vi "LC Transfer.vi"(8 "error in (no error)":errorcluster caption="Error In", 9 "Value In":string, 10 "Property":string, 11 "Ctl Ref In":refnum<vi>) -> (0 "error out":errorcluster caption="Error Out", 1 "Value Out":string, 3 "Ctl Ref Out":refnum<vi>)   [LabVIEW 2020]
uses:
  <vilib>/Utility/miscctls.llb/LVOutOfRangeActionTypeDef.ctl
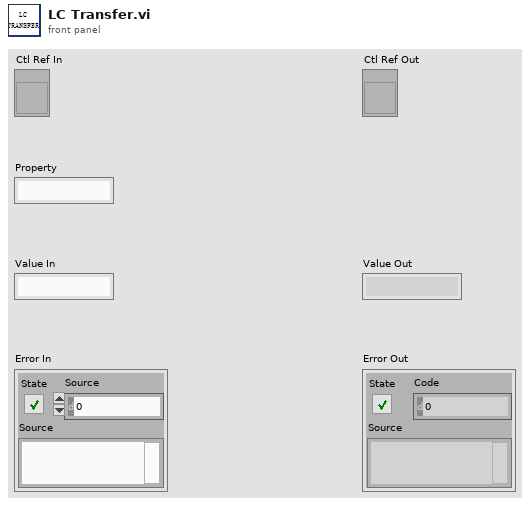
[diagram p1: front panel]
types:
  T1 = typedef "LVPositionTypeDef.ctl" = cluster{"Left":i32, "Top":i32}
  T2 = typedef "LVOutOfRangeActionTypeDef.ctl" = cluster{"Out of Range Action Minimum":u8, "Out of Range Action Maximum":u8, "Out of Range Action Increment":u8}
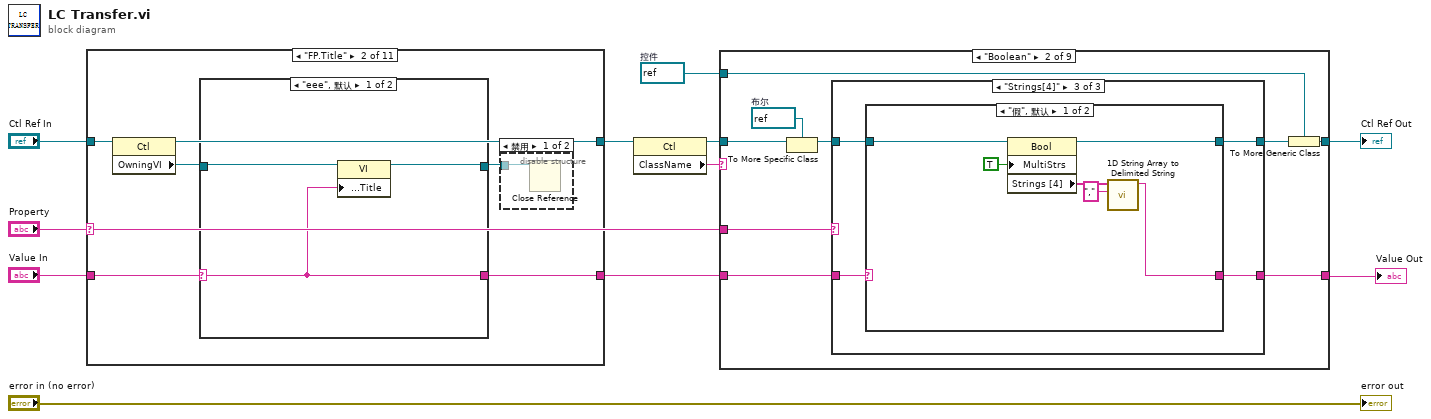
[diagram p0: block diagram]
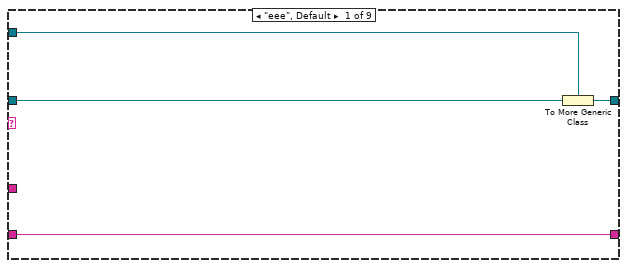
[diagram p2: hidden frame]
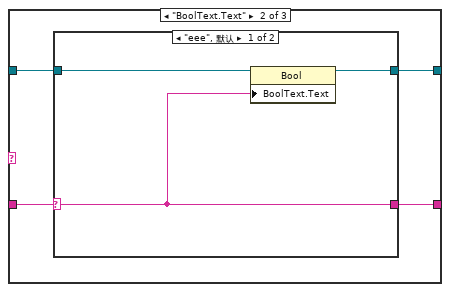
[diagram p4: hidden frame]
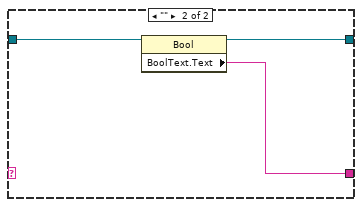
[diagram p5: hidden frame]
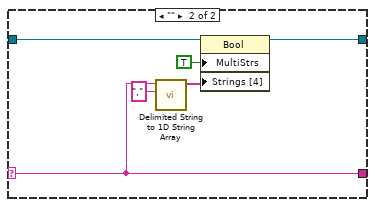
[diagram p6: hidden frame]
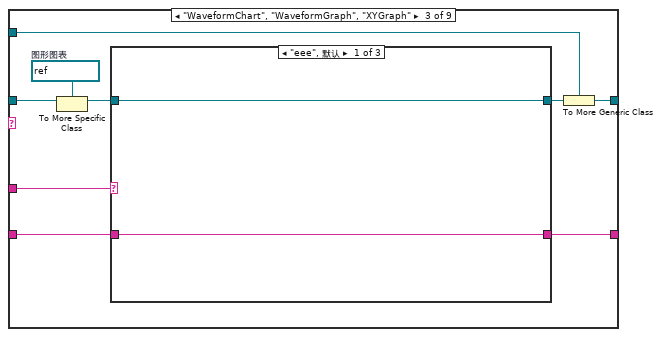
[diagram p7: hidden frame]
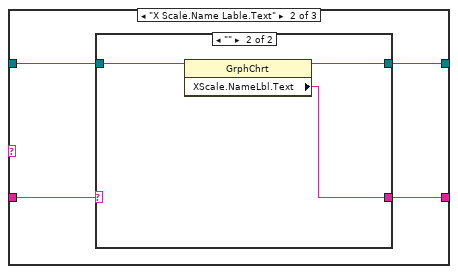
[diagram p8: hidden frame]
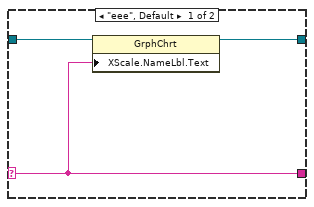
[diagram p9: hidden frame]
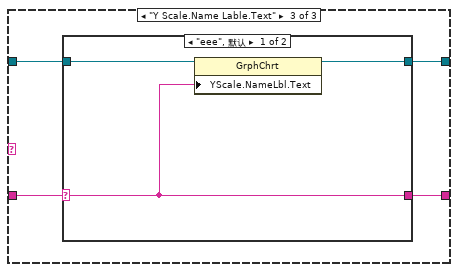
[diagram p10: hidden frame]
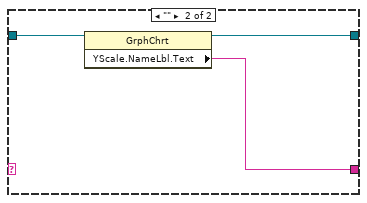
[diagram p11: hidden frame]
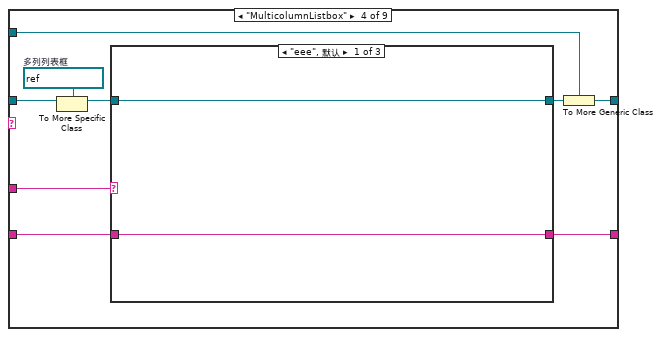
[diagram p12: hidden frame]
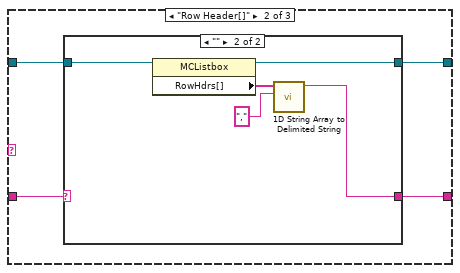
[diagram p13: hidden frame]
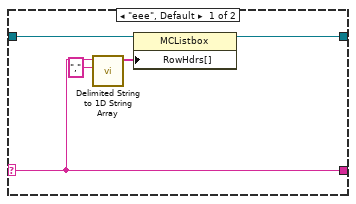
[diagram p14: hidden frame]
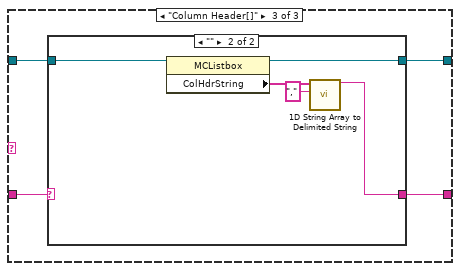
[diagram p15: hidden frame]
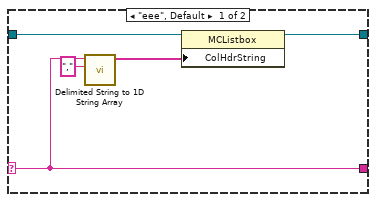
[diagram p16: hidden frame]
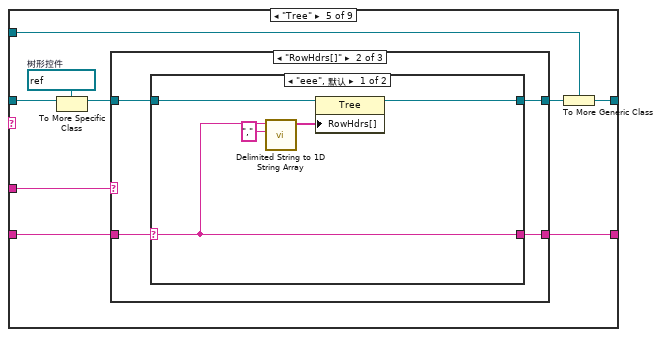
[diagram p17: hidden frame]
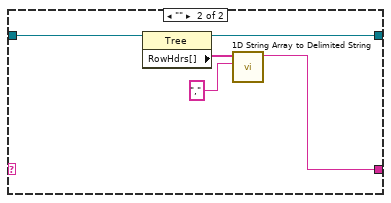
[diagram p19: hidden frame]
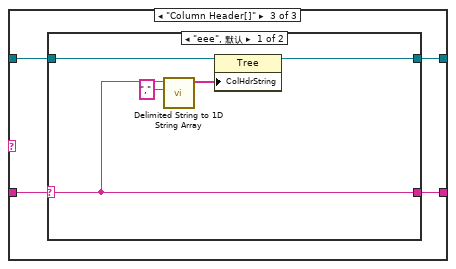
[diagram p20: hidden frame]
diagram:
  w10 = refnum<vi> refnum  # 控件
  n1 = case shown="\"FP.Title\"" "Property" {
    tunnel: [w13 w18 w27 w38 w48 w59 w75 w91 w107 w123 w146] -> w11
    tunnel: "Ctl Ref In" -> [w13 w19 w29 w40 w50 w60 w76 w92 w108 w124 w147]
    tunnel: "Value In" -> [w12 w15 w30 w39 w49 w58 w74 w90 w106 w122 w145]
    tunnel: [w12 w14 w28 w37 w47 w57 w73 w89 w105 w121 w144] -> w9
    frame "eee", Default {
    }
    frame "FP.Title" {
      n2 = property class="Ctl"(reference=w19) -> (reference out=w18:refnum<vi>, "OwningVI"=w17:refnum<vi>)  [unwired: 1 in, 1 out]
      n3 = case shown="\"eee\", 默认" w15 {
        selector: w15 -> [w21 _]
        tunnel: w17 -> [w23 w26]
        tunnel: [w22 w25] -> w16
        tunnel: [w21 w24] -> w14
        frame "eee", Default {
          n4 = property class="VI"(reference=w23, "Front Panel.Title"=w21) -> (reference out=w22:refnum<vi>)  [unwired: 1 in, 1 out]
        }
        frame "" {
          n5 = property class="VI"(reference=w26) -> (reference out=w25:refnum<vi>, "Front Panel.Title"=w24:string)  [unwired: 1 in, 1 out]
        }
      }
      n6 = disable-structure shown="禁用" {
        disable-tunnel: w16 -> [w20 _]
        frame Disabled {
          n7 = Close Reference(reference=w20) -> ()  [unwired: 1 in, 1 out]
        }
        frame Enabled {
        }
      }
    }
    frame "Lable.Text" {
      n8 = case shown="\"eee\", 默认" w30 {
        selector: w30 -> [w31 _]
        tunnel: w29 -> [w33 w36]
        tunnel: [w31 w35] -> w28
        tunnel: [w32 w34] -> w27
        frame "eee", Default {
          n9 = property class="Ctl"(reference=w33, "Label.Text"=w31) -> (reference out=w32:refnum<vi>)  [unwired: 1 in, 1 out]
        }
        frame "" {
          n10 = property class="Ctl"(reference=w36) -> (reference out=w34:refnum<vi>, "Label.Text"=w35:string)  [unwired: 1 in, 1 out]
        }
      }
    }
    frame "Desc" {
      n11 = case shown="\"eee\", 默认" w39 {
        selector: w39 -> [w41 _]
        tunnel: w40 -> [w43 w46]
        tunnel: [w42 w45] -> w38
        tunnel: [w41 w44] -> w37
        frame "eee", Default {
          n12 = property class="Ctl"(reference=w43, "Desc"=w41) -> (reference out=w42:refnum<vi>)  [unwired: 1 in, 1 out]
        }
        frame "" {
          n13 = property class="Ctl"(reference=w46) -> (reference out=w45:refnum<vi>, "Desc"=w44:string)  [unwired: 1 in, 1 out]
        }
      }
    }
    frame "TipStrip" {
      n14 = case shown="\"eee\", 默认" w49 {
        selector: w49 -> [w51 _]
        tunnel: w50 -> [w53 w56]
        tunnel: [w52 w55] -> w48
        tunnel: [w51 w54] -> w47
        frame "eee", Default {
          n15 = property class="Ctl"(reference=w53, "TipStrip"=w51) -> (reference out=w52:refnum<vi>)  [unwired: 1 in, 1 out]
        }
        frame "" {
          n16 = property class="Ctl"(reference=w56) -> (reference out=w55:refnum<vi>, "TipStrip"=w54:string)  [unwired: 1 in, 1 out]
        }
      }
    }
    frame "Visible" {
      n17 = case shown="\"eee\", 默认" w58 {
        selector: w58 -> [_ w67]
        tunnel: w60 -> [w66 w72]
        tunnel: [w65 w71] -> w59
        tunnel: [w61 w67] -> w57
        frame "eee", Default {
          n18 = property class="Ctl"(reference=w66) -> (reference out=w65:refnum<vi>, "Visible"=w64:bool)  [unwired: 1 in, 1 out]
          n19 = Select(t="1", s=w64, f="0") -> (s? t:f=w61:string)
        }
        frame "" {
          n20 = call <vilib>:"Trim Whitespace.vi"("string"=w67) -> ("trimmed string"=w70:string)  [unwired: 1 in]
          n21 = Decimal String To Number(string=w70) -> (number=w69:i32)  [unwired: 2 in, 1 out]
          n22 = Greater Than 0?(x=w69) -> (x > 0?=w68:bool)
          n23 = property class="Ctl"(reference=w72, "Visible"=w68) -> (reference out=w71:refnum<vi>)  [unwired: 1 in, 1 out]
        }
      }
    }
    frame "Caption.Visible" {
      n24 = case shown="\"eee\", 默认" w74 {
        selector: w74 -> [w77 _]
        tunnel: w76 -> [w82 w88]
        tunnel: [w81 w83] -> w75
        tunnel: [w77 w84] -> w73
        frame "eee", Default {
          n25 = call <vilib>:"Trim Whitespace.vi"("string"=w77) -> ("trimmed string"=w80:string)  [unwired: 1 in]
          n26 = Decimal String To Number(string=w80) -> (number=w79:i32)  [unwired: 2 in, 1 out]
          n27 = Greater Than 0?(x=w79) -> (x > 0?=w78:bool)
          n28 = property class="Ctl"(reference=w82, "Caption.Visible"=w78) -> (reference out=w81:refnum<vi>)  [unwired: 1 in, 1 out]
        }
        frame "" {
          n29 = property class="Ctl"(reference=w88) -> (reference out=w83:refnum<vi>, "Caption.Visible"=w87:bool)  [unwired: 1 in, 1 out]
          n30 = Select(t="1", s=w87, f="0") -> (s? t:f=w84:string)
        }
      }
    }
    frame "Lable.Visible" {
      n31 = case shown="\"eee\", 默认" w90 {
        selector: w90 -> [w93 _]
        tunnel: w92 -> [w98 w104]
        tunnel: [w97 w99] -> w91
        tunnel: [w93 w100] -> w89
        frame "eee", Default {
          n32 = call <vilib>:"Trim Whitespace.vi"("string"=w93) -> ("trimmed string"=w96:string)  [unwired: 1 in]
          n33 = Decimal String To Number(string=w96) -> (number=w95:i32)  [unwired: 2 in, 1 out]
          n34 = Greater Than 0?(x=w95) -> (x > 0?=w94:bool)
          n35 = property class="Ctl"(reference=w98, "Label.Visible"=w94) -> (reference out=w97:refnum<vi>)  [unwired: 1 in, 1 out]
        }
        frame "" {
          n36 = property class="Ctl"(reference=w104) -> (reference out=w99:refnum<vi>, "Label.Visible"=w103:bool)  [unwired: 1 in, 1 out]
          n37 = Select(t="1", s=w103, f="0") -> (s? t:f=w100:string)
        }
      }
    }
    frame "Blinking" {
      n38 = case shown="\"eee\", 默认" w106 {
        selector: w106 -> [w109 _]
        tunnel: w108 -> [w114 w120]
        tunnel: [w113 w119] -> w107
        tunnel: [w109 w115] -> w105
        frame "eee", Default {
          n39 = call <vilib>:"Trim Whitespace.vi"("string"=w109) -> ("trimmed string"=w112:string)  [unwired: 1 in]
          n40 = Decimal String To Number(string=w112) -> (number=w111:i32)  [unwired: 2 in, 1 out]
          n41 = Greater Than 0?(x=w111) -> (x > 0?=w110:bool)
          n42 = property class="Ctl"(reference=w114, "Blinking"=w110) -> (reference out=w113:refnum<vi>)  [unwired: 1 in, 1 out]
        }
        frame "" {
          n43 = property class="Ctl"(reference=w120) -> (reference out=w119:refnum<vi>, "Blinking"=w118:bool)  [unwired: 1 in, 1 out]
          n44 = Select(t="1", s=w118, f="0") -> (s? t:f=w115:string)
        }
      }
    }
    frame "Caption.Position" {
      n45 = case shown="\"\"" w122 {
        selector: w122 -> [w125 _]
        tunnel: w124 -> [w133 w143]
        tunnel: [w132 w134] -> w123
        tunnel: [w125 w135] -> w121
        frame "eee", Default {
          n46 = call <vilib>:"Delimited String to 1D String Array.vi"("delimiter"=",", "delimited string"=w125) -> ("string array"=w130:string[])  [unwired: 9 in]
          n47 = Fract/Exp String To Number(string=w130) -> (number=w129:dbl[])  [unwired: 3 in, 1 out]
          n48 = Index Array(array=w129) -> (element #1=w128:dbl, element #2=w127:dbl)  [unwired: 2 in]
          n49 = Bundle("String"=w128, "String"=w127) -> (w126:cluster{"String":dbl, "String":dbl})  [unwired: 1 in]
          n50 = property class="Ctl"(reference=w133, "Caption.Position"=w126) -> (reference out=w132:refnum<vi>)  [unwired: 1 in, 1 out]
        }
        frame "" {
          n51 = property class="Ctl"(reference=w143) -> (reference out=w134:refnum<vi>, "Caption.Position"=w142:T1)  [unwired: 1 in, 1 out]
          n52 = Unbundle(w142) -> ("Left"=w141:i32, "Top"=w140:i32)
          n53 = Build Array(w141, w140) -> (w139:i32[])
          n54 = Number To Fractional String(number=w139, precision (6)=i16 0 ("精度(6)")) -> (F-format string=w137:string[])  [unwired: 2 in]
          n55 = call <vilib>:"1D String Array to Delimited String.vi"("delimiter"=",", "string array"=w137) -> ("delimited string"=w135:string)  [unwired: 9 in]
        }
      }
    }
    frame "Caption.Text" {
      n56 = case shown="\"eee\", 默认" w145 {
        selector: w145 -> [w148 _]
        tunnel: w147 -> [w152 w155]
        tunnel: [w151 w154] -> w146
        tunnel: [w148 w153] -> w144
        frame "eee", Default {
          n57 = property class="Ctl"(reference=w152, "Caption.Visible"=TRUE ("可见"), "Caption.Text"=w148, "Label.Visible"=FALSE ("标签.可见")) -> (reference out=w151:refnum<vi>)  [unwired: 1 in, 1 out]
        }
        frame "" {
          n58 = property class="Ctl"(reference=w155, "Visible"=TRUE ("可见")) -> (reference out=w154:refnum<vi>, "Caption.Text"=w153:string)  [unwired: 1 in, 1 out]
        }
      }
    }
  }
  n59 = property class="Ctl"(reference=w11) -> (reference out=w4:refnum<vi>, "ClassName"=w3:string)  [unwired: 1 in, 1 out]
  n60 = case shown="\"Boolean\"" w3 {
    tunnel: "Property" -> [_ w169 w205 w236 w275 w314 w339 w387 w433]
    tunnel: w4 -> [w160 w168 w206 w237 w276 w315 w340 w389 w434]
    tunnel: [w159 w164 w204 w235 w274 w313 w338 w383 w430] -> w5
    tunnel: w10 -> [w158 w163 w203 w234 w273 w312 w337 w382 _]
    tunnel: w9 -> [w157 w162 w199 w230 w270 w308 w333 w384 w432]
    tunnel: [w157 w161 w198 w229 w268 w307 w332 w381 w429] -> w2
    frame "eee", Default {
      n61 = To More Generic Class(target class=w158, reference=w160) -> (generic class reference=w159:refnum<vi>)
    }
    frame "Boolean" {
      w166 = refnum<vi> refnum  # 布尔
      n62 = To More Specific Class(target class=w166, reference=w168) -> (specific class reference=w167:refnum<vi>)  [unwired: 1 in, 1 out]
      n63 = case shown="\"Strings[4]\"" w169 {
        tunnel: w167 -> [w171 w175 w185]
        tunnel: [w171 w174 w184] -> w165
        tunnel: w162 -> [w170 w173 w183]
        tunnel: [w170 w172 w182] -> w161
        frame "eee", Default {
        }
        frame "BoolText.Text" {
          n64 = case shown="\"eee\", 默认" w173 {
            selector: w173 -> [w176 _]
            tunnel: w175 -> [w178 w181]
            tunnel: [w177 w180] -> w174
            tunnel: [w176 w179] -> w172
            frame "eee", Default {
              n65 = property class="Bool"(reference=w178, "BoolText.Text"=w176) -> (reference out=w177:refnum<vi>)  [unwired: 1 in, 1 out]
            }
            frame "" {
              n66 = property class="Bool"(reference=w181) -> (reference out=w180:refnum<vi>, "BoolText.Text"=w179:string)  [unwired: 1 in, 1 out]
            }
          }
        }
        frame "Strings[4]" {
          n67 = case shown="\"假\", 默认" w183 {
            selector: w183 -> [_ w192]
            tunnel: w185 -> [w191 w196]
            tunnel: [w190 w195] -> w184
            tunnel: [w186 w192] -> w182
            frame "假", Default {
              n68 = property class="Bool"(reference=w191, "MultiStrs"=TRUE ("多文本字符串")) -> (reference out=w190:refnum<vi>, "Strings [4]"=w188:string[])  [unwired: 1 in, 1 out]
              n69 = call <vilib>:"1D String Array to Delimited String.vi"("delimiter"=",", "string array"=w188) -> ("delimited string"=w186:string)  [unwired: 9 in]
            }
            frame "" {
              n70 = call <vilib>:"Delimited String to 1D String Array.vi"("delimiter"=",", "delimited string"=w192) -> ("string array"=w193:string[])  [unwired: 9 in]
              n71 = property class="Bool"(reference=w196, "MultiStrs"=TRUE ("多文本字符串"), "Strings [4]"=w193) -> (reference out=w195:refnum<vi>)  [unwired: 1 in, 1 out]
            }
          }
        }
      }
      n72 = To More Generic Class(target class=w163, reference=w165) -> (generic class reference=w164:refnum<vi>)
    }
    frame "WaveformChart", "WaveformGraph", "XYGraph" {
      w200 = refnum<vi> refnum  # 图形图表
      n73 = To More Specific Class(target class=w200, reference=w206) -> (specific class reference=w202:refnum<vi>)  [unwired: 1 in, 1 out]
      n74 = case shown="\"eee\", 默认" w205 {
        tunnel: w202 -> [w208 w212 w222]
        tunnel: [w208 w211 w221] -> w201
        tunnel: w199 -> [w207 w210 w220]
        tunnel: [w207 w209 w219] -> w198
        frame "eee", Default {
        }
        frame "X Scale.Name Lable.Text" {
          n75 = case shown="\"\"" w210 {
            selector: w210 -> [w213 _]
            tunnel: w212 -> [w215 w218]
            tunnel: [w214 w217] -> w211
            tunnel: [w213 w216] -> w209
            frame "eee", Default {
              n76 = property class="GrphChrt"(reference=w215, "XScale.NameLbl.Text"=w213) -> (reference out=w214:refnum<vi>)  [unwired: 1 in, 1 out]
            }
            frame "" {
              n77 = property class="GrphChrt"(reference=w218) -> (reference out=w217:refnum<vi>, "XScale.NameLbl.Text"=w216:string)  [unwired: 1 in, 1 out]
            }
          }
        }
        frame "Y Scale.Name Lable.Text" {
          n78 = case shown="\"eee\", 默认" w220 {
            selector: w220 -> [w223 _]
            tunnel: w222 -> [w225 w228]
            tunnel: [w224 w227] -> w221
            tunnel: [w223 w226] -> w219
            frame "eee", Default {
              n79 = property class="GrphChrt"(reference=w225, "YScale.NameLbl.Text"=w223) -> (reference out=w224:refnum<vi>)  [unwired: 1 in, 1 out]
            }
            frame "" {
              n80 = property class="GrphChrt"(reference=w228) -> (reference out=w227:refnum<vi>, "YScale.NameLbl.Text"=w226:string)  [unwired: 1 in, 1 out]
            }
          }
        }
      }
      n81 = To More Generic Class(target class=w203, reference=w201) -> (generic class reference=w204:refnum<vi>)
    }
    frame "MulticolumnListbox" {
      w231 = refnum<vi> refnum  # 多列列表框
      n82 = To More Specific Class(target class=w231, reference=w237) -> (specific class reference=w233:refnum<vi>)  [unwired: 1 in, 1 out]
      n83 = case shown="\"eee\", 默认" w236 {
        tunnel: w233 -> [w239 w243 w257]
        tunnel: [w239 w242 w256] -> w232
        tunnel: w230 -> [w238 w241 w255]
        tunnel: [w238 w240 w254] -> w229
        frame "eee", Default {
        }
        frame "Row Header[]" {
          n84 = case shown="\"\"" w241 {
            selector: w241 -> [w244 _]
            tunnel: w243 -> [w248 w253]
            tunnel: [w247 w252] -> w242
            tunnel: [w244 w249] -> w240
            frame "eee", Default {
              n85 = call <vilib>:"Delimited String to 1D String Array.vi"("delimiter"=",", "delimited string"=w244) -> ("string array"=w245:string[])  [unwired: 9 in]
              n86 = property class="MCListbox"(reference=w248, "RowHdrs[]"=w245) -> (reference out=w247:refnum<vi>)  [unwired: 1 in, 1 out]
            }
            frame "" {
              n87 = property class="MCListbox"(reference=w253) -> (reference out=w252:refnum<vi>, "RowHdrs[]"=w251:string[])  [unwired: 1 in, 1 out]
              n88 = call <vilib>:"1D String Array to Delimited String.vi"("delimiter"=",", "string array"=w251) -> ("delimited string"=w249:string)  [unwired: 9 in]
            }
          }
        }
        frame "Column Header[]" {
          n89 = case shown="\"\"" w255 {
            selector: w255 -> [w258 _]
            tunnel: w257 -> [w262 w267]
            tunnel: [w261 w266] -> w256
            tunnel: [w258 w263] -> w254
            frame "eee", Default {
              n90 = call <vilib>:"Delimited String to 1D String Array.vi"("delimiter"=",", "delimited string"=w258) -> ("string array"=w259:string[])  [unwired: 9 in]
              n91 = property class="MCListbox"(reference=w262, "ColHdrString"=w259) -> (reference out=w261:refnum<vi>)  [unwired: 1 in, 1 out]
            }
            frame "" {
              n92 = property class="MCListbox"(reference=w267) -> (reference out=w266:refnum<vi>, "ColHdrString"=w265:string[])  [unwired: 1 in, 1 out]
              n93 = call <vilib>:"1D String Array to Delimited String.vi"("delimiter"=",", "string array"=w265) -> ("delimited string"=w263:string)  [unwired: 9 in]
            }
          }
        }
      }
      n94 = To More Generic Class(target class=w234, reference=w232) -> (generic class reference=w235:refnum<vi>)
    }
    frame "Tree" {
      w269 = refnum<vi> refnum  # 树形控件
      n95 = To More Specific Class(target class=w269, reference=w276) -> (specific class reference=w272:refnum<vi>)  [unwired: 1 in, 1 out]
      n96 = case shown="\"RowHdrs[]\"" w275 {
        tunnel: w272 -> [w278 w282 w296]
        tunnel: [w278 w281 w295] -> w271
        tunnel: w270 -> [w277 w280 w294]
        tunnel: [w277 w279 w293] -> w268
        frame "eee", Default {
        }
        frame "RowHdrs[]" {
          n97 = case shown="\"eee\", 默认" w280 {
            selector: w280 -> [w283 _]
            tunnel: w282 -> [w287 w292]
            tunnel: [w286 w291] -> w281
            tunnel: [w283 w288] -> w279
            frame "eee", Default {
              n98 = call <vilib>:"Delimited String to 1D String Array.vi"("delimiter"=",", "delimited string"=w283) -> ("string array"=w284:string[])  [unwired: 9 in]
              n99 = property class="Tree"(reference=w287, "RowHdrs[]"=w284) -> (reference out=w286:refnum<vi>)  [unwired: 1 in, 1 out]
            }
            frame "" {
              n100 = property class="Tree"(reference=w292) -> (reference out=w291:refnum<vi>, "RowHdrs[]"=w290:string[])  [unwired: 1 in, 1 out]
              n101 = call <vilib>:"1D String Array to Delimited String.vi"("delimiter"=",", "string array"=w290) -> ("delimited string"=w288:string)  [unwired: 9 in]
            }
          }
        }
        frame "Column Header[]" {
          n102 = case shown="\"eee\", 默认" w294 {
            selector: w294 -> [w297 _]
            tunnel: w296 -> [w301 w306]
            tunnel: [w300 w304] -> w295
            tunnel: [w297 w302] -> w293
            frame "eee", Default {
              n103 = call <vilib>:"Delimited String to 1D String Array.vi"("delimiter"=",", "delimited string"=w297) -> ("string array"=w298:string[])  [unwired: 9 in]
              n104 = property class="Tree"(reference=w301, "ColHdrString"=w298) -> (reference out=w300:refnum<vi>)  [unwired: 1 in, 1 out]
            }
            frame "" {
              n105 = property class="Tree"(reference=w306) -> (reference out=w304:refnum<vi>, "ColHdrString"=w305:string[])  [unwired: 1 in, 1 out]
              n106 = call <vilib>:"1D String Array to Delimited String.vi"("delimiter"=",", "string array"=w305) -> ("delimited string"=w302:string)  [unwired: 9 in]
            }
          }
        }
      }
      n107 = To More Generic Class(target class=w273, reference=w271) -> (generic class reference=w274:refnum<vi>)
    }
    frame "Ring" {
      w309 = refnum<vi> refnum  # 下拉列表
      n108 = To More Specific Class(target class=w309, reference=w315) -> (specific class reference=w311:refnum<vi>)  [unwired: 1 in, 1 out]
      n109 = case shown="\"Strings[]\"" w314 {
        tunnel: w311 -> [w317 w321]
        tunnel: [w317 w320] -> w310
        tunnel: w308 -> [w316 w319]
        tunnel: [w316 w318] -> w307
        frame "eee", Default {
        }
        frame "Strings[]" {
          n110 = case shown="\"eee\", 默认" w319 {
            selector: w319 -> [w322 _]
            tunnel: w321 -> [w326 w331]
            tunnel: [w325 w330] -> w320
            tunnel: [w322 w327] -> w318
            frame "eee", Default {
              n111 = call <vilib>:"Delimited String to 1D String Array.vi"("delimiter"="*****", "delimited string"=w322) -> ("string array"=w323:string[])  [unwired: 9 in]
              n112 = property class="Ring"(reference=w326, "Strings []"=w323) -> (reference out=w325:refnum<vi>)  [unwired: 1 in, 1 out]
            }
            frame "" {
              n113 = property class="Ring"(reference=w331) -> (reference out=w330:refnum<vi>, "Strings []"=w329:string[])  [unwired: 1 in, 1 out]
              n114 = call <vilib>:"1D String Array to Delimited String.vi"("delimiter"="*****", "string array"=w329) -> ("delimited string"=w327:string)  [unwired: 9 in]
            }
          }
        }
      }
      n115 = To More Generic Class(target class=w312, reference=w310) -> (generic class reference=w313:refnum<vi>)
    }
    frame "String" {
      w334 = refnum<vi> refnum  # 字符串
      n116 = To More Specific Class(target class=w334, reference=w340) -> (specific class reference=w336:refnum<vi>)  [unwired: 1 in, 1 out]
      n117 = case shown="\"Text.Text\"" w339 {
        tunnel: w336 -> [w342 w346 w356 w371]
        tunnel: [w342 w345 w355 w370] -> w335
        tunnel: w333 -> [w341 w344 w354 w369]
        tunnel: [w341 w343 w353 w368] -> w332
        frame "eee", Default {
        }
        frame "Text.Text" {
          n118 = case shown="\"eee\", 默认" w344 {
            selector: w344 -> [w347 _]
            tunnel: w346 -> [w349 w352]
            tunnel: [w348 w351] -> w345
            tunnel: [w347 w350] -> w343
            frame "eee", Default {
              n119 = property class="Str"(reference=w349, "Text.Text"=w347) -> (reference out=w348:refnum<vi>)  [unwired: 1 in, 1 out]
            }
            frame "" {
              n120 = property class="Str"(reference=w352) -> (reference out=w351:refnum<vi>, "Text.Text"=w350:string)  [unwired: 1 in, 1 out]
            }
          }
        }
        frame "FondBold" {
          n121 = case shown="\"\"" w354 {
            selector: w354 -> [w357 _]
            tunnel: w356 -> [w359 w367]
            tunnel: [w358 w366] -> w355
            tunnel: [w357 w362] -> w353
            frame "eee", Default {
              n122 = Equal?(x=w357, y="1") -> (x = y?=w360:bool)
              n123 = property class="Str"(reference=w359, "Text.FontBold"=w360) -> (reference out=w358:refnum<vi>)  [unwired: 1 in, 1 out]
            }
            frame "" {
              n124 = property class="Str"(reference=w367) -> (reference out=w366:refnum<vi>, "Text.FontBold"=w365:bool)  [unwired: 1 in, 1 out]
              n125 = Select(t="1", s=w365, f="") -> (s? t:f=w362:string)
            }
          }
        }
        frame "TextColor" {
          n126 = case shown="\"eee\", 默认" w369 {
            selector: w369 -> [w372 _]
            tunnel: w371 -> [w374 w380]
            tunnel: [w373 w379] -> w370
            tunnel: [w372 w377] -> w368
            frame "eee", Default {
              n127 = call <vilib>:"Trim Whitespace.vi"("string"=w372) -> ("trimmed string"=w376:string)  [unwired: 1 in]
              n128 = Hexadecimal String To Number(string=w376) -> (number=w375:u32)  [unwired: 2 in, 1 out]
              n129 = property class="Str"(reference=w374, "Text.TextColor"=w375) -> (reference out=w373:refnum<vi>)  [unwired: 1 in, 1 out]
            }
            frame "" {
              n130 = property class="Str"(reference=w380) -> (reference out=w379:refnum<vi>, "Text.TextColor"=w378:u32)  [unwired: 1 in, 1 out]
              n131 = Number To Hexadecimal String(2:w378) -> (0:w377:string)  [unwired: 1 in]
            }
          }
        }
      }
      n132 = To More Generic Class(target class=w337, reference=w335) -> (generic class reference=w338:refnum<vi>)
    }
    frame "Numenic" {
      w388 = refnum<vi> refnum  # 数字
      n133 = To More Specific Class(target class=w388, reference=w389) -> (specific class reference=w386:refnum<vi>)  [unwired: 1 in, 1 out]
      n134 = case shown="\"eee\", 默认" w387 {
        tunnel: w386 -> [w391 w395 w404]
        tunnel: [w391 w394 w405] -> w385
        tunnel: w384 -> [w390 w393 w403]
        tunnel: [w390 w392 w402] -> w381
        frame "eee", Default {
        }
        frame "FormatString" {
          n135 = case shown="\"eee\", 默认" w393 {
            selector: w393 -> [w396 _]
            tunnel: w395 -> [w398 w401]
            tunnel: [w397 w400] -> w394
            tunnel: [w396 w399] -> w392
            frame "eee", Default {
              n136 = property class="DigNum"(reference=w398, "FormatString"=w396) -> (reference out=w397:refnum<vi>)  [unwired: 1 in, 1 out]
            }
            frame "" {
              n137 = property class="DigNum"(reference=w401) -> (reference out=w400:refnum<vi>, "FormatString"=w399:string)  [unwired: 1 in, 1 out]
            }
          }
        }
        frame "DataEntryLimits" {
          n138 = case shown="\"\"" w403 {
            selector: w403 -> [w406 _]
            tunnel: [w408 w417] -> w405
            tunnel: w404 -> [w407 w425]
            tunnel: [w406 w418] -> w402
            frame "eee", Default {
              n139 = call <vilib>:"Trim Whitespace.vi"("string"=w406) -> ("trimmed string"=w415:string)  [unwired: 1 in]
              n140 = call <vilib>:"Delimited String to 1D String Array.vi"("delimiter"="," ("split"), "delimited string"=w415) -> ("string array"=w413:string[])  [unwired: 9 in]
              n141 = Fract/Exp String To Number(string=w413) -> (number=w412:dbl[])  [unwired: 3 in, 1 out]
              n142 = Index Array(array=w412) -> (element #1=w411:dbl, element #2=w410:dbl, element #3=w409:dbl)  [unwired: 3 in]
              n143 = property class="DigNum"(reference=w407, "Minimum"=w411, "Maximum"=w410, "Increment"=w409, "OutOfRngAction"=T2 {"Out of Range Action Minimum"=1, "Out of Range Action Maximum"=1, "Out of Range Action Increment"=1} ("Response to Value Outside Limits")) -> (reference out=w408:refnum<vi>)  [unwired: 1 in, 1 out]
            }
            frame "" {
              n144 = property class="DigNum"(reference=w425) -> (reference out=w417:refnum<vi>, "Minimum"=w423:dbl, "Maximum"=w424:dbl, "Increment"=w422:dbl)  [unwired: 1 in, 1 out]
              n145 = Build Array(w423, w424, w422) -> (w421:dbl[])
              n146 = for {
                tunnel: w421 -> [w428] mode=indexing
                tunnel: [w426] -> w420 mode=indexing
                n147 = Format Into String(format string="%#.6f" ("格式字符串"), w428) -> (resulting string=w426:string)  [unwired: 2 in, 1 out]
              }
              n148 = call <vilib>:"1D String Array to Delimited String.vi"("delimiter"=",", "string array"=w420) -> ("delimited string"=w418:string)  [unwired: 9 in]
            }
          }
        }
      }
      n149 = To More Generic Class(target class=w382, reference=w385) -> (generic class reference=w383:refnum<vi>)
    }
    frame "Combox" {
      w435 = refnum<vi> refnum  # 组合框
      n150 = To More Specific Class(target class=w435, reference=w434) -> (specific class reference=w431:refnum<vi>)  [unwired: 1 in, 1 out]
      n151 = case shown="\"Strings[]\"" w433 {
        tunnel: w432 -> [w436 w439]
        tunnel: w431 -> [w437 w441]
        tunnel: [w437 w440] -> w430
        tunnel: [w436 w438] -> w429
        frame "eee", Default {
        }
        frame "Strings[]" {
          n152 = case shown="\"eee\", 默认" w439 {
            selector: w439 -> [w442 _]
            tunnel: w441 -> [w446 w451]
            tunnel: [w445 w450] -> w440
            tunnel: [w442 w447] -> w438
            frame "eee", Default {
              n153 = call <vilib>:"Delimited String to 1D String Array.vi"("delimiter"="*****", "delimited string"=w442) -> ("string array"=w444:string[])  [unwired: 9 in]
              n154 = property class="CmbBox"(reference=w446, "Strings[]"=w444) -> (reference out=w445:refnum<vi>)  [unwired: 1 in, 1 out]
            }
            frame "" {
              n155 = property class="CmbBox"(reference=w451) -> (reference out=w450:refnum<vi>, "Strings[]"=w449:string[])  [unwired: 1 in, 1 out]
              n156 = call <vilib>:"1D String Array to Delimited String.vi"("delimiter"="*****", "string array"=w449) -> ("delimited string"=w447:string)  [unwired: 9 in]
            }
          }
        }
      }
    }
  }
  "Ctl Ref Out" <- w5
  "Value Out" <- w2
  "error out" <- "error in (no error)"
